vi "ADC Stop Continue Read.vi"(11 "DevHandle":i32) -> (3 "function return":i32)   [LabVIEW 2010, in "usb2adc.lvlib"]
doc: "int WINAPI ADC_StopContinueRead(int DevHandle);"
uses:
  usb2adc.lvlib
  USB2XXX.dll
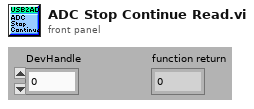
[diagram p1: front panel]
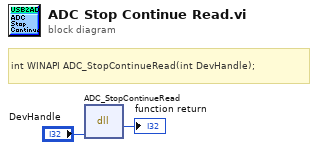
[diagram p0: block diagram]
diagram:
  # "int WINAPI ADC_StopContinueRead(int DevHandle);"
  n1 = dll-call lib="G:/OtherWork/USB2XXX_Example/trunk/Labview/PublicFiles/usb2adc/USB2XXX.*" fn="ADC_StopContinueRead"("DevHandle"="DevHandle") -> (→"function return":i32)  [unwired: 4 in, 2 out]
